vi "Exec2017.vi"(8 "Commands in":string) -> (3 "Commands out":string, 4 "Missing parameters":bool)   [LabVIEW 2017]
uses:
  <vilib>/regexp/Match Regular Expression.xnode
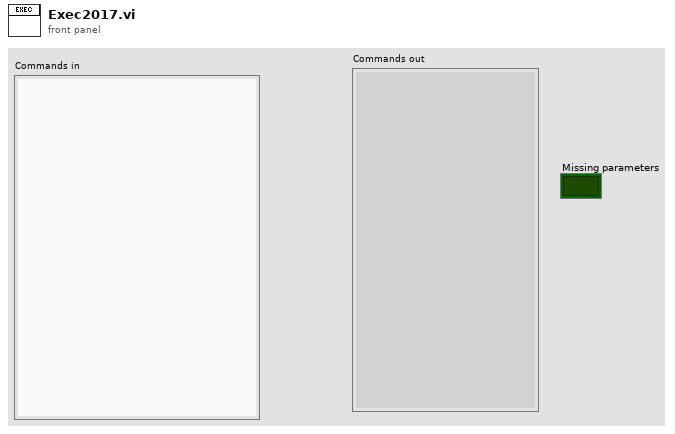
[diagram p1: front panel]
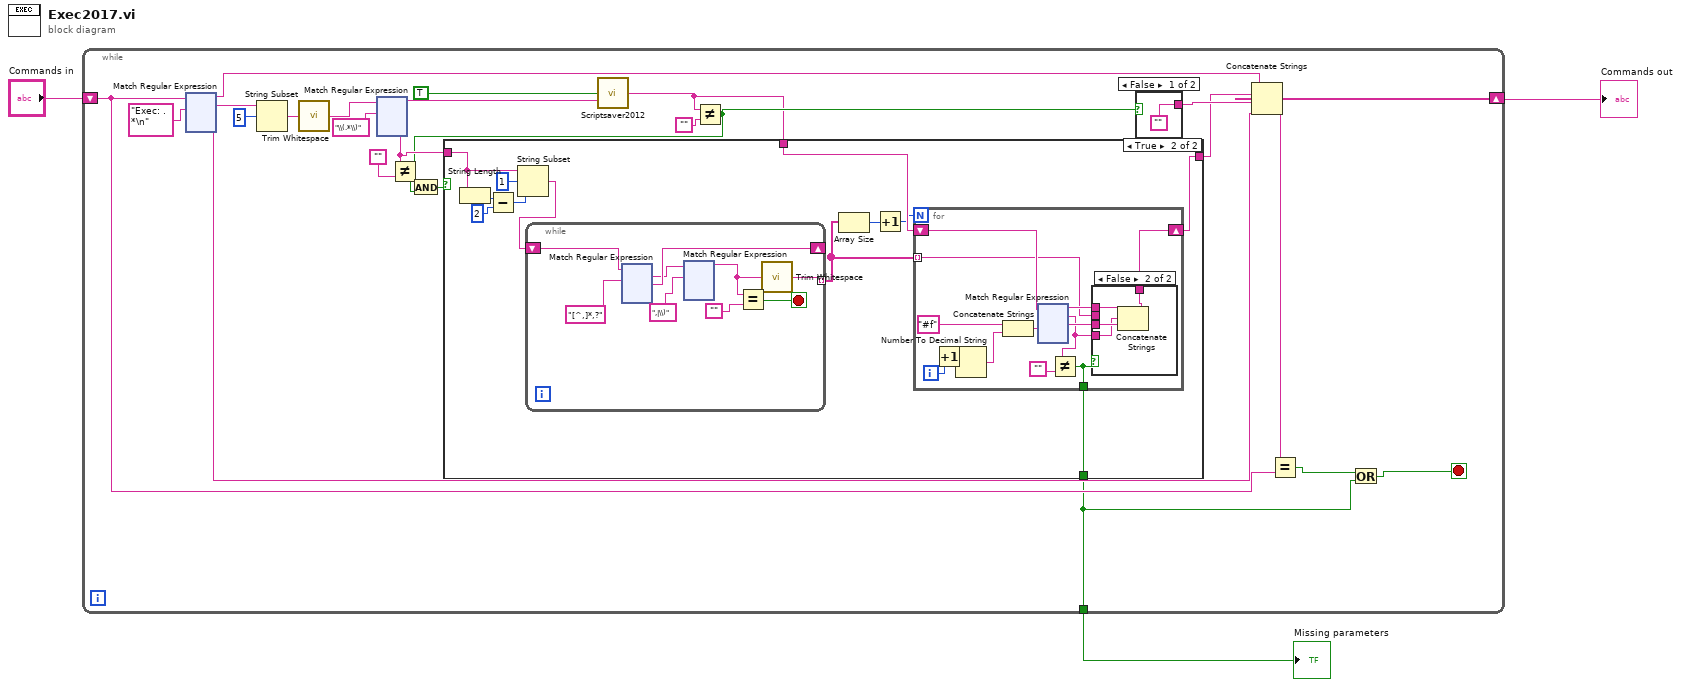
[diagram p0: block diagram]
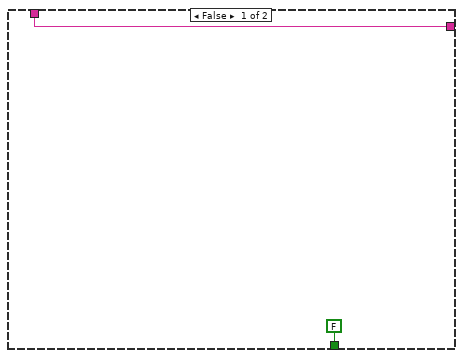
[diagram p2: hidden frame]
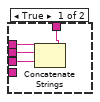
[diagram p3: hidden frame]
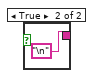
[diagram p4: hidden frame]
diagram:
  n1 = while {
    shift-right: [w19] -> w2
    shift-left: "Commands in" -> [w18]
    tunnel: [w4] -> w1
    stop <- w5 stop-if-true
    n2 = xnode "Match Regular Expression"("input string"=w18, "regular expression"="Exec: .*\n") -> ("before match"=w23:string, "whole match"=w26:string, "after match"=w21:string)  [unwired: 4 in, 2 out]
    n3 = String Subset(string=w26, offset (0)=5) -> (substring=w22:string)  [unwired: 1 in]
    n4 = call <vilib>:"Trim Whitespace.vi"("string"=w22) -> ("trimmed string"=w16:string)  [unwired: 1 in]
    n5 = xnode "Match Regular Expression"("input string"=w16, "regular expression"="\\(.*\\)") -> ("before match"=w14:string, "whole match"=w12:string)  [unwired: 4 in, 3 out]
    n6 = Not Equal?(x=w12, y="") -> (x != y?=w11:bool)
    n7 = call "Scriptsaver2012.vi"("Filename"=w14, "Save (0)/Load (1)"=TRUE) -> ("Loaded Script"=w8:string)  [unwired: 1 in]
    n8 = Not Equal?(x=w8, y="") -> (x != y?=w10:bool)
    n9 = And(x=w10, y=w11) -> (x .and. y?=w9:bool)
    n10 = case shown="True" w9 {
      tunnel: w12 -> [_ w35]
      tunnel: w8 -> [w29 w40]
      tunnel: [w29 w39] -> w7
      tunnel: [FALSE w30] -> w4
      frame False {
      }
      frame True {
        n11 = String Length(string=w35) -> (length=w38:i32)
        n12 = Subtract(x=w38, y=2) -> (x-y=w36:i32)
        n13 = String Subset(string=w35, offset (0)=1, length (rest)=w36) -> (substring=w33:string)
        n14 = while {
          tunnel: [w178] -> w41 mode=indexing
          shift-right: [w183] -> _
          shift-left: w33 -> [w184]
          stop <- w181 stop-if-true
          n15 = xnode "Match Regular Expression"("input string"=w184, "regular expression"="[^,]*,?") -> ("whole match"=w179:string, "after match"=w183:string)  [unwired: 4 in, 3 out]
          n16 = xnode "Match Regular Expression"("input string"=w179, "regular expression"=",|\\)") -> ("before match"=w177:string)  [unwired: 4 in, 4 out]
          n17 = Equal?(x=w177, y="") -> (x = y?=w181:bool)
          n18 = call <vilib>:"Trim Whitespace.vi"("string"=w177) -> ("trimmed string"=w178:string)  [unwired: 1 in]
        }
        n19 = Array Size(array=w41) -> (size(s)=w32:i32)
        n20 = Increment(x=w32) -> (x+1=w31:i32)
        n21 = for {
          N: w31 -> [_]
          tunnel: w41 -> [w46] mode=indexing
          shift-right: [w45] -> w39
          shift-left: w40 -> [w49]
          tunnel: [w43] -> w30
          i -> [w52]
          n22 = Increment(x=w52) -> (x+1=w51:i32)
          n23 = Number To Decimal String(number=w51) -> (decimal integer string=w54:string)  [unwired: 1 in]
          n24 = Concatenate Strings("#f" ("string"), w54) -> (w50:string)
          n25 = xnode "Match Regular Expression"("input string"=w49, "regular expression"=w50) -> ("before match"=w48:string, "whole match"=w42:string, "after match"=w47:string)  [unwired: 4 in, 2 out]
          n26 = Not Equal?(x=w42, y="") -> (x != y?=w43:bool)
          n27 = case shown="False" w43 {
            tunnel: w48 -> [w58 w62]
            tunnel: w47 -> [w57 w61]
            tunnel: w46 -> [w56 _]
            tunnel: [w55 w60] -> w45
            tunnel: w42 -> [_ w59]
            frame True {
              n28 = Concatenate Strings(w58, w56, w57) -> (w55:string)
            }
            frame False {
              n29 = Concatenate Strings(w62, w59, w61) -> (w60:string)
            }
          }
        }
      }
    }
    n30 = case shown="False" w10 {
      tunnel: ["" "\n"] -> w20
      frame False {
      }
      frame True {
      }
    }
    n31 = Concatenate Strings(w23, w7, w20, w21) -> (w19:string)
    n32 = Equal?(x=w19, y=w18) -> (x = y?=w6:bool)
    n33 = Or(x=w6, y=w4) -> (x .or. y?=w5:bool)
  }
  "Commands out" <- w2
  "Missing parameters" <- w1
